vi "write32.vi"(8 "error out":errorcluster caption="error in", 9 "起始地址":u32, 10 "U32":u32[](array[numeric]), 11 "VISA资源名称输入":refnum<visa-resource-name>) -> (0 "error out 2":errorcluster caption="error out", 3 "VISA资源名称输出":refnum<visa-resource-name>)   [LabVIEW 2012]
uses:
  <vilib>/Instr/_visa.llb/VISA Register Access Address Space.ctl
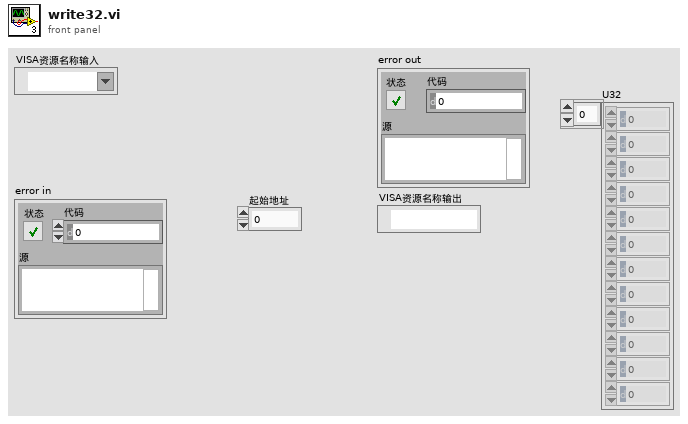
[diagram p1: front panel]
types:
  T1 = typedef "VISA Register Access Address Space.ctl" = u16
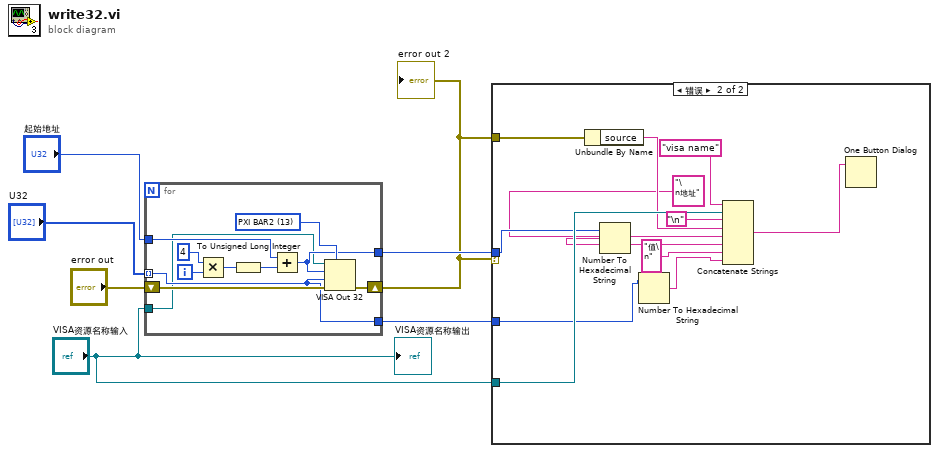
[diagram p0: block diagram]
diagram:
  n1 = for {
    tunnel: "U32" -> [w9] mode=indexing
    tunnel: "起始地址" -> [w18]
    shift-right: [w15] -> w2
    shift-left: "error out" -> [w14]
    tunnel: [w10] -> w4
    tunnel: [w9] -> w3
    tunnel: "VISA资源名称输入" -> [w8]
    i -> [w17]
    w12 = T1 13 items=["VXI/VME A16"=1, "VXI/VME A24"=2, "VXI/VME A32"=3, "VXI/VME A64"=4, "PXI内存分配"=9, "PXI配置"=10, "PXI BAR0"=11, "PXI BAR1"=12, "PXI BAR2"=13, "PXI BAR3"=14, "PXI BAR4"=15, "PXI BAR5"=16] ("Address Space")
    n2 = Multiply(x=4, y=w17) -> (x*y=w13:i32)
    n3 = To Unsigned Long Integer(number=w13) -> (unsigned 32bit integer=w11:u32)
    n4 = Add(x=w18, y=w11) -> (x+y=w10:u32)
    n5 = VISA Out 32(7:w12, 8:w14, 9:w9, 10:w10, 11:w8) -> (0:w15:errorcluster)  [unwired: 1 out]
  }
  "error out 2" <- w2
  n6 = case shown="错误" w2 {
    tunnel: "VISA资源名称输入" -> [_ w30]
    tunnel: w2 -> [_ w29]
    tunnel: w4 -> [_ w27]
    tunnel: w3 -> [_ w26]
    frame No Error {
    }
    frame Error {
      n7 = Unbundle By Name(w29) -> ("source"=w28:string)
      n8 = Number To Hexadecimal String(2:w27) -> (0:w24:string)  [unwired: 1 in]
      n9 = Number To Hexadecimal String(2:w26) -> (0:w22:string)  [unwired: 1 in]
      n10 = Concatenate Strings("visa name" ("字符串"), w30, "\n", w28, "\n地址" ("字符串"), w24, "值\n" ("字符串"), w22) -> (w21:string)
      n11 = One Button Dialog(message=w21) -> ()  [unwired: 1 in, 1 out]
    }
  }
  "VISA资源名称输出" <- "VISA资源名称输入"
